vi "ke37xx Configure Channel Specifier.vi"(0 "VISA Resource Name":refnum<visa-resource-name>, 1 "Column":string, 2 "Index":string, 5 "Slot":u8=1 min=1 max=6 step=1, 7 "Bank":string, 9 "Row":string, 11 "error in (no error)":errorcluster, 12 "Backplane":string) -> (4 "VISA Resource Name Out":refnum<visa-resource-name>, 8 "Channel String":string, 15 "error out":errorcluster)   [LabVIEW 2009, in "Keithley 3700 Series.lvlib"]
doc: "This VI returns an appropriate channel designation string based on various physical attributes, such as slot, row, col, bank, index or backplane. Inputs that are accepted are based upon the type of card in the specified slot.\n\nThere are 5 valid input combinations to this vi, other input combinations are invalid:\n\n1: <slot>, <bank>, <row>, <column>\n2: <slot>, <row>, <column>\n3: <slot>, <bank>, <index>\n4: <slot>, <index>\n5: <slot>, <backplane> \n\nType of card in slot Function variants to use\n---------------------------------------------------------------------------\nMatrix card containing banks Variant 1 or 5\nMatrix card without banks Variant 2 or 5\nMultiplexer cards Variant 3, 4, or 5\n\n\nFor example, the following code creates a channel for a 3724 card in slot 2, Bank 2, Index 1:\n\ncd = createspecifier(2, 2, 1)\nprint(cd)\n2031"
uses:
  <instrlib>/Keithley 3706/Keithley 3700 Series.lvlib
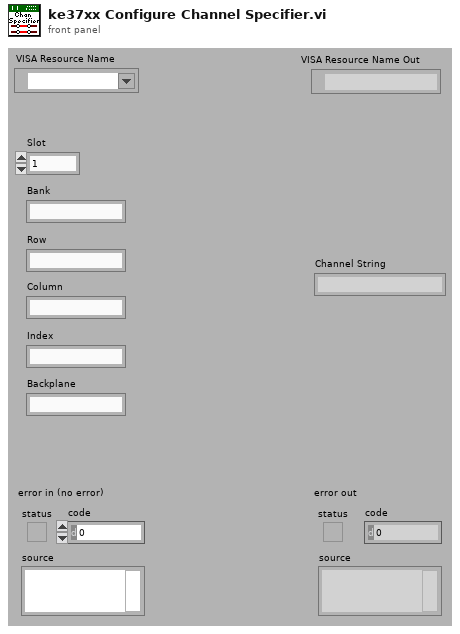
[diagram p1: front panel]
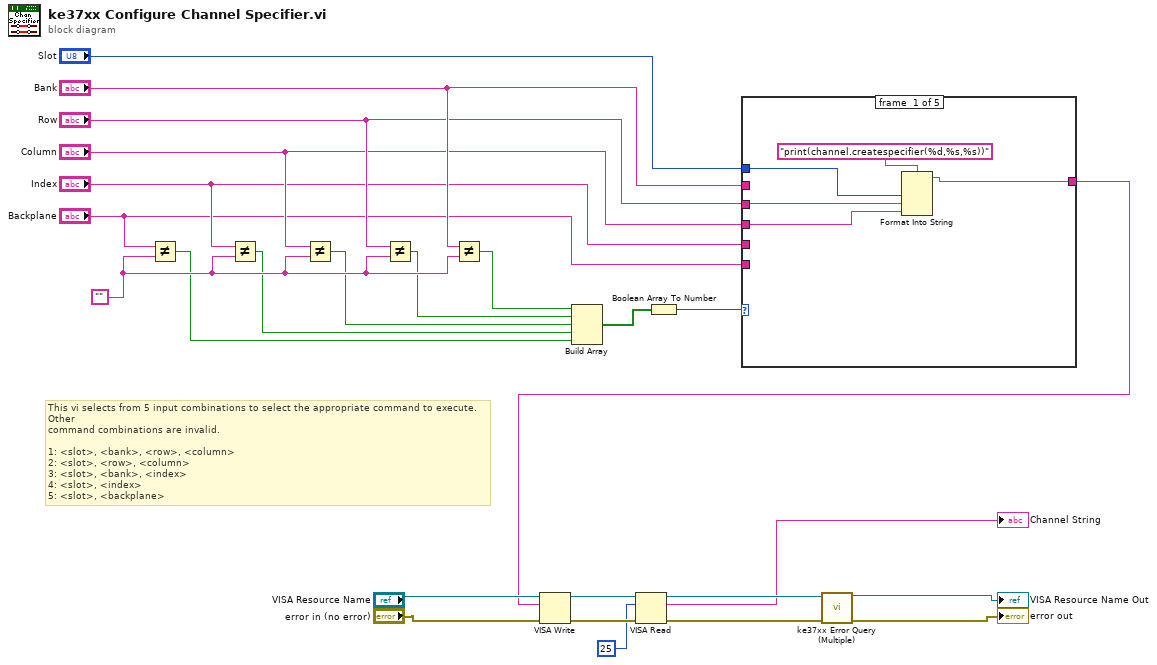
[diagram p0: block diagram]
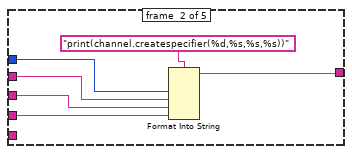
[diagram p2: hidden frame]
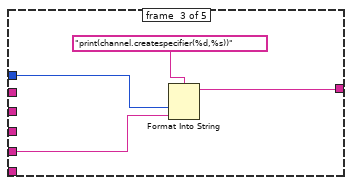
[diagram p3: hidden frame]
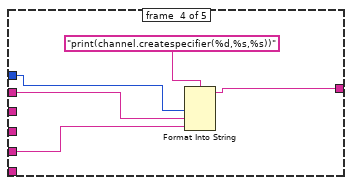
[diagram p4: hidden frame]
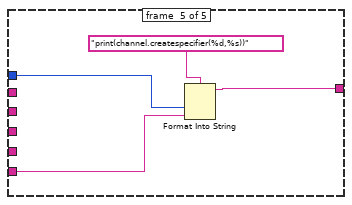
[diagram p5: hidden frame]
diagram:
  w15 = ""
  # "This vi selects from 5 input combinations to select the appropriate command to execute. Other\ncommand combinations are invalid.\n\n1: <slot>, <bank>, <row>, <column>\n2: <slot>, <row>, <column>\n3: <slot>, <bank>, <index>\n4: <slot>, <index>\n5: <slot>, <backplane>"
  n1 = Not Equal?(x="Backplane", y=w15) -> (x != y?=w10:bool)
  n2 = Not Equal?(x="Index", y=w15) -> (x != y?=w11:bool)
  n3 = Not Equal?(x="Column", y=w15) -> (x != y?=w12:bool)
  n4 = Not Equal?(x="Row", y=w15) -> (x != y?=w13:bool)
  n5 = Not Equal?(x="Bank", y=w15) -> (x != y?=w14:bool)
  n6 = Build Array(w14, w13, w12, w11, w10) -> (w9:bool[])
  n7 = Boolean Array To Number(Boolean array=w9) -> (number=w8:u32)
  n8 = case shown="6" w8 {
    tunnel: "Slot" -> [w30 w36 w39 w44 w48]
    tunnel: "Bank" -> [_ w35 _ w43 _]
    tunnel: "Row" -> [w27 w34 _ _ _]
    tunnel: "Column" -> [w29 w33 _ _ _]
    tunnel: "Index" -> [_ _ w38 w42 _]
    tunnel: "Backplane" -> [_ _ _ _ w47]
    tunnel: [w26 w31 w37 w41 w46] -> w1
    frame #0 {
      n9 = Format Into String(format string="print(channel.createspecifier(%d,%s,%s))", w30, w27, w29) -> (resulting string=w26:string)  [unwired: 2 in, 1 out]
    }
    frame #1 {
      n10 = Format Into String(format string="print(channel.createspecifier(%d,%s,%s,%s))", w36, w35, w34, w33) -> (resulting string=w31:string)  [unwired: 2 in, 1 out]
    }
    frame #2 {
      n11 = Format Into String(format string="print(channel.createspecifier(%d,%s))", w39, w38) -> (resulting string=w37:string)  [unwired: 2 in, 1 out]
    }
    frame #3 {
      n12 = Format Into String(format string="print(channel.createspecifier(%d,%s,%s))", w44, w43, w42) -> (resulting string=w41:string)  [unwired: 2 in, 1 out]
    }
    frame #4 {
      n13 = Format Into String(format string="print(channel.createspecifier(%d,%s))", w48, w47) -> (resulting string=w46:string)  [unwired: 2 in, 1 out]
    }
  }
  n14 = VISA Write(VISA resource name="VISA Resource Name", write buffer=w1, error in (no error)="error in (no error)") -> (VISA resource name out=w25:refnum<visa-resource-name>, error out=w24:errorcluster)  [unwired: 1 out]
  n15 = VISA Read(VISA resource name=w25, byte count=25, error in (no error)=w24) -> (VISA resource name out=w22:refnum<visa-resource-name>, read buffer=→"Channel String":string, error out=w23:errorcluster)  [unwired: 1 out]
  n16 = call <instrlib>:"ke37xx Error Query (Multiple).vi"("VISA resource name"=w22, "error in (no error)"=w23) -> ("VISA resource name out"=→"VISA Resource Name Out":refnum<visa-resource-name>, "error out"=→"error out":errorcluster)  [unwired: 12 out]
